vi "Global 1.vi"() -> ()   [LabVIEW 2012]
panel:
  in  "Current RPM":dbl
  in  "RPM?":bool
  in  "Goal RPM":dbl
  in  "Output Power":dbl
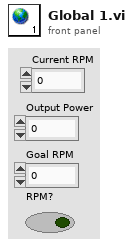
[diagram p1: front panel]
diagram:
